vi "findCurrentSetpoint.vi"(7 "Initial Timestamp":timestamp, 9 "Current Timestamp":timestamp, 10 "Setpoint Profile":cluster{"time (s)":dbl, "setpoint":dbl}[](array[cluster])) -> (2 "Setpoint":dbl)   [LabVIEW 2018]
panel:
  out "Current Stage":dbl
  out "Relative Time":dbl
  # "Given an initial timestamp, a current timestamp, and a setpoint profile, this program will calculate the\ncurrent setpoint expected from the controller"
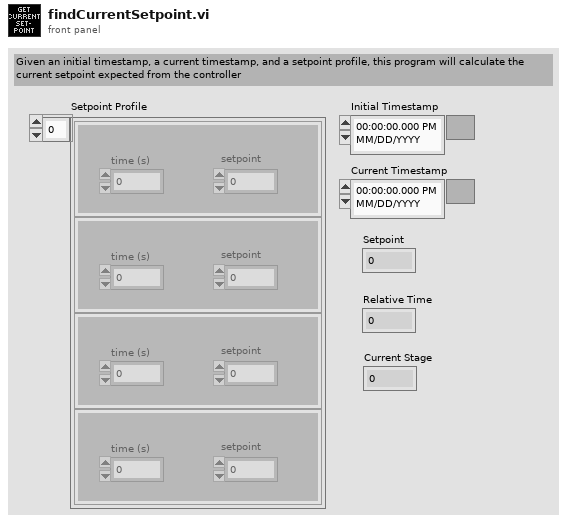
[diagram p1: front panel]
types:
  T1 = cluster{"time buffer":dbl, "setpoint buffer":dbl}
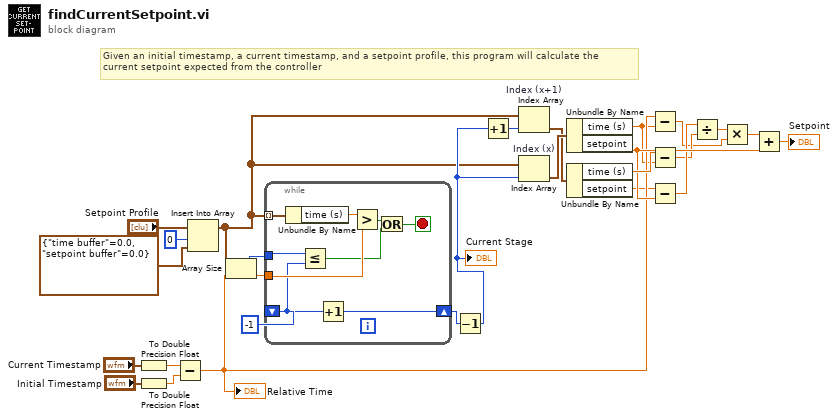
[diagram p0: block diagram]
diagram:
  # "Given an initial timestamp, a current timestamp, and a setpoint profile, this program will calculate the\ncurrent setpoint expected from the controller"
  n1 = To Double Precision Float(number="Current Timestamp") -> (double precision float=w15:dbl)
  n2 = To Double Precision Float(number="Initial Timestamp") -> (double precision float=w16:dbl)
  n3 = Subtract(x=w15, y=w16) -> (x-y=w10:dbl)
  "Relative Time" <- w10
  n4 = Insert Into Array(array="Setpoint Profile", index=0, new element=T1 {"time buffer"=0.0, "setpoint buffer"=0.0}) -> (w2:cluster{"time (s)":dbl, "setpoint":dbl}[])
  n5 = Array Size(array=w2) -> (size(s)=w1:i32)
  n6 = while {
    tunnel: w10 -> [w33]
    tunnel: w2 -> [w35] mode=indexing
    shift-right: [w34] -> w4
    shift-left: -1 -> [w30]
    tunnel: w1 -> [w31]
    stop <- w27 stop-if-true
    n7 = Unbundle By Name(w35) -> ("time (s)"=w32:dbl)
    n8 = Less Or Equal?(x=w31, y=w30) -> (x <= y?=w29:bool)
    n9 = Increment(x=w30) -> (x+1=w34:i32)
    n10 = Greater?(x=w32, y=w33) -> (0:w28:bool)
    n11 = Or(x=w28, y=w29) -> (x .or. y?=w27:bool)
  }
  n12 = Decrement(x=w4) -> (x-1=w3:i32)
  "Current Stage" <- w3
  n13 = Increment(x=w3) -> (x+1=w21:i32)
  n14 = Index Array "Index (x+1)"(array=w2, index=w21) -> (element=w6:cluster{"time (s)":dbl, "setpoint":dbl})
  n15 = Index Array "Index (x)"(array=w2, index=w3) -> (element=w7:cluster{"time (s)":dbl, "setpoint":dbl})
  n16 = Unbundle By Name(w7) -> ("time (s)"=w8:dbl, "setpoint"=w18:dbl)
  n17 = Unbundle By Name(w6) -> ("time (s)"=w20:dbl, "setpoint"=w9:dbl)
  n18 = Subtract(x=w10, y=w8) -> (x-y=w11:dbl)
  n19 = Subtract(x=w20, y=w8) -> (x-y=w13:dbl)
  n20 = Subtract(x=w9, y=w18) -> (x-y=w14:dbl)
  n21 = Divide(x=w14, y=w13) -> (x/y=w12:dbl)
  n22 = Multiply(x=w12, y=w11) -> (x*y=w19:dbl)
  n23 = Add(x=w19, y=w18) -> (x+y=→"Setpoint":dbl)
